vi "Get Bucket Website.vi"(8 "error in (no error)":errorcluster, 11 "Bucket in":refnum<class "Bucket.lvclass">) -> (0 "error out":errorcluster, 2 "Website Configuration":T1, 3 "Bucket out":refnum<class "Bucket.lvclass">)   [LabVIEW 2015, in "NI_AWS_S3.lvlib" / "Bucket.lvclass"]
uses:
  Bucket.lvclass
  Website Configuration.ctl
  Core/HTTP Request/Region handling.ctl
  Core/HTTP Request/Name Value Pair.ctl
  Core/HTTP Request/Request Options.ctl
  Core/HTTP Request/URL formatting.ctl
  Bucket.lvclass/Bucket.ctl
  Read Name.vi
  Core/HTTP Request/HTTP Request.lvclass
  NI_AWS_S3.lvlib
  XML Parsing/NI_XML Parsing.lvlib
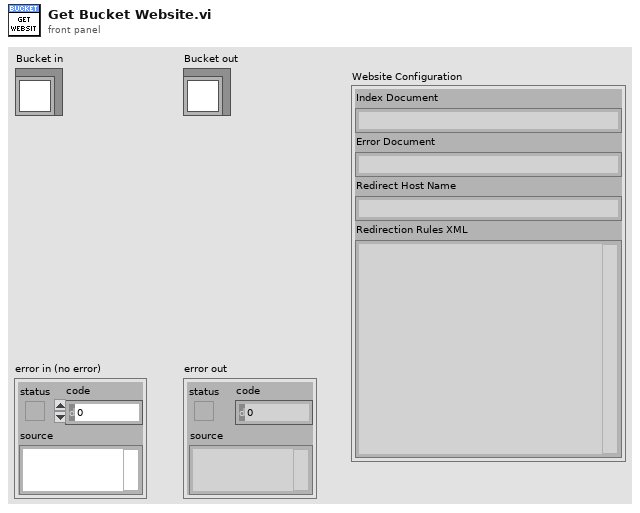
[diagram p1: front panel]
types:
  T1 = typedef "NI_AWS_S3.lvlib/Website Configuration.ctl" = cluster{"Index Document":string, "Error Document":string, "Redirect Host Name":string, "Redirection Rules XML":string}
  T2 = typedef "NI_AWS_Core.lvlib/HTTP Request.lvclass/Request Options.ctl" = cluster{"request headers":T3[], "request parameters":T3[], "request body":string, "region handling":T4, "URL formatting":T5}
  T3 = typedef "NI_AWS_Core.lvlib/HTTP Request.lvclass/Name Value Pair.ctl" = cluster{"name":string, "value":string}
  T4 = typedef "NI_AWS_Core.lvlib/HTTP Request.lvclass/Region handling.ctl" = enum16{"use region everywhere", "use region (authentication only)", "use region (URL only)", "ignore region everwhere"}
  T5 = typedef "NI_AWS_Core.lvlib/HTTP Request.lvclass/URL formatting.ctl" = enum16{"region-", "region."}
  T6 = typedef "NI_AWS_Core.lvlib/HTTP Request.lvclass/Response.ctl" = cluster{"Headers":string, "Body":string}
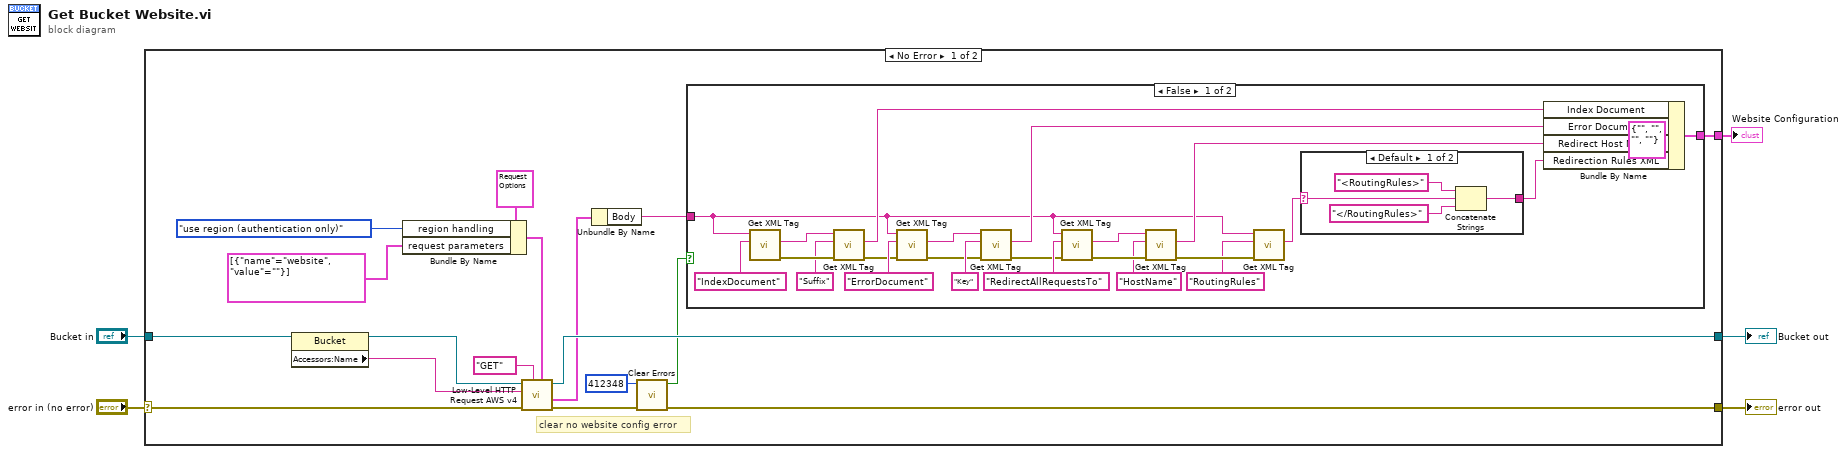
[diagram p0: block diagram]
diagram:
  n1 = case shown="No Error" "error in (no error)" {
    selector: "error in (no error)" -> [w18 w52]
    tunnel: "Bucket in" -> [w19 w51]
    tunnel: [w11 w52] -> w3
    tunnel: [w12 w51] -> w2
    tunnel: [w7 _] -> w1
    frame No Error {
      # "clear no website config error"
      n2 = property class="Bucket"(reference=w19) -> (reference out=w13:refnum<class "Bucket.lvclass">, "Accessors:Name"=w22:string)  [unwired: 1 in, 1 out]
      n3 = Bundle By Name(cluster=T2 {"request headers"=[], "request parameters"=[], "request body"="", "region handling"=enum."use region everywhere", "URL formatting"=enum."region."} ("Request Options"), "region handling"=Region_handling."use region (authentication only)", "request parameters"=T3[] [{"name"="website", "value"=""}]) -> (w14:T2)
      n4 = call "Low-Level HTTP Request AWS v4.vi"("Request Options"=w14, "HTTP-Verb"="GET", "error in (no error)"=w18, "URL Prefix"=w22, "AWS Core in"=w13) -> ("error out"=w17:errorcluster, "Response"=w9:T6, "AWS Core out"=w12:refnum<class "Bucket.lvclass">)  [unwired: 3 in, 1 out]
      n5 = Unbundle By Name(w9) -> ("Body"=w8:string)
      n6 = call <vilib>:"Clear Errors.vi"("error in (no error)"=w17, "specific error code to clear (0: all)"=412348) -> ("error out"=w11:errorcluster, "specific error cleared?"=w6:bool)  [unwired: 4 in]
      n7 = case shown="False" w6 {
        tunnel: w8 -> [w25 _]
        tunnel: [w23 _] -> w7
        frame False {
          n8 = call "Get XML Tag.vi"("Tag name"="IndexDocument", "XML String in"=w25) -> ("error out"=w45:errorcluster, "Tag value"=w44:string)  [unwired: 5 in, 3 out]
          n9 = call "Get XML Tag.vi"("error in (no error)"=w45, "Tag name"="Suffix", "XML String in"=w44) -> ("error out"=w37:errorcluster, "Tag value"=w42:string)  [unwired: 4 in, 3 out]
          n10 = call "Get XML Tag.vi"("error in (no error)"=w37, "Tag name"="ErrorDocument", "XML String in"=w25) -> ("error out"=w39:errorcluster, "Tag value"=w40:string)  [unwired: 4 in, 3 out]
          n11 = call "Get XML Tag.vi"("error in (no error)"=w39, "Tag name"="Key", "XML String in"=w40) -> ("error out"=w31:errorcluster, "Tag value"=w36:string)  [unwired: 4 in, 3 out]
          n12 = call "Get XML Tag.vi"("error in (no error)"=w31, "Tag name"="RedirectAllRequestsTo", "XML String in"=w25) -> ("error out"=w34:errorcluster, "Tag value"=w33:string)  [unwired: 4 in, 3 out]
          n13 = call "Get XML Tag.vi"("error in (no error)"=w34, "Tag name"="HostName", "XML String in"=w33) -> ("error out"=w29:errorcluster, "Tag value"=w30:string)  [unwired: 4 in, 3 out]
          n14 = call "Get XML Tag.vi"("error in (no error)"=w29, "Tag name"="RoutingRules", "XML String in"=w25) -> ("Tag value"=w27:string)  [unwired: 4 in, 4 out]
          n15 = case shown="Default" w27 {
            selector: w27 -> [w50 _]
            tunnel: [w49 _] -> w26
            frame Default {
              n16 = Concatenate Strings("<RoutingRules>", w50, "</RoutingRules>") -> (w49:string)
            }
            frame "" {
            }
          }
          n17 = Bundle By Name(cluster=T1 {"Index Document"="", "Error Document"="", "Redirect Host Name"="", "Redirection Rules XML"=""} ("Website Configuration"), "Index Document"=w42, "Error Document"=w36, "Redirect Host Name"=w30, "Redirection Rules XML"=w26) -> (w23:T1)
        }
        frame True {
        }
      }
    }
    frame Error {
    }
  }
  "error out" <- w3
  "Bucket out" <- w2
  "Website Configuration" <- w1
